vi "split.vi"(10 "长度":i32=4, 11 "source":string) -> (2 "left":string, 3 "right":string)   [LabVIEW 2011]
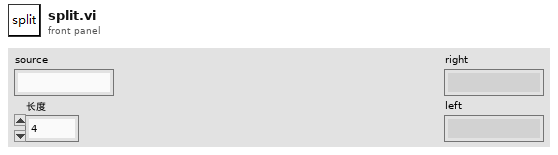
[diagram p1: front panel]
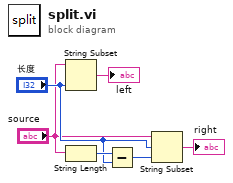
[diagram p0: block diagram]
diagram:
  n1 = String Subset(string="source", length (rest)="长度") -> (substring=→"left":string)  [unwired: 1 in]
  n2 = String Length(string="source") -> (length=w6:i32)
  n3 = Subtract(x=w6, y="长度") -> (x-y=w4:i32)
  n4 = String Subset(string="source", offset (0)="长度", length (rest)=w4) -> (substring=→"right":string)
